vi "Set_Horizontal_ROI.vi"(8 "error in (no error)":errorcluster, 10 "input cluster":T1={"Mode"=enum."ROI", "Manual LUT"={"Minimum"=0.0, "Maximum"=0.0}, "ImageProcessed"=refnum, "Image "=refnum, "Log?"=FALSE, "Auto?"=FALSE, "ROI"={"Global Rectangle"=[], "Contours"=[]}, "ROI Parameters"={"Count"=0.0, "Size(um)"=0.0}, "Image X"=0, "Image Y"=0, "Horizontal ROI"={"Global Rectangle"=[], "Contours"=[]}, "HROI Pos"=0, "Custom ROI"={"Global Rectangle"=[], "Contours"=[]}, "Intensity Graph"=[], "Image Type"=7} {"Image Type" items=["Grayscale (U8)", "Grayscale (U16)"]; "ROI Parameters"."Size(um)" min=0 max=255 step=0.1 format="%.2f"; "ROI Parameters"."Count" min=0 max=255 step=0.1 format="%.2f"}) -> (0 "error out":errorcluster, 2 "output cluster":T1={"Mode"=enum."ROI", "Manual LUT"={"Minimum"=0.0, "Maximum"=0.0}, "ImageProcessed"=refnum, "Image "=refnum, "Log?"=FALSE, "Auto?"=FALSE, "ROI"={"Global Rectangle"=[], "Contours"=[]}, "ROI Parameters"={"Count"=0.0, "Size(um)"=0.0}, "Image X"=0, "Image Y"=0, "Horizontal ROI"={"Global Rectangle"=[], "Contours"=[]}, "HROI Pos"=0, "Custom ROI"={"Global Rectangle"=[], "Contours"=[]}, "Intensity Graph"=[], "Image Type"=7} {"Image Type" items=["Grayscale (U8)", "Grayscale (U16)"]; "ROI Parameters"."Size(um)" min=0 max=255 step=0.1 format="%.2f"; "ROI Parameters"."Count" min=0 max=255 step=0.1 format="%.2f"})   [LabVIEW 2023, in "Camera_Controller.lvlib"]
uses:
  Camera_Controller.lvlib
  typedefs/ImageProcessingParameters.ctl
  <vilib>/vision/Image Controls.llb/IMAQ Image.ctl
  typedefs/Image Type.ctl
  <vilib>/vision/NI_Vision_Development_Module.lvlib
  typedefs/typedefs.lvlib
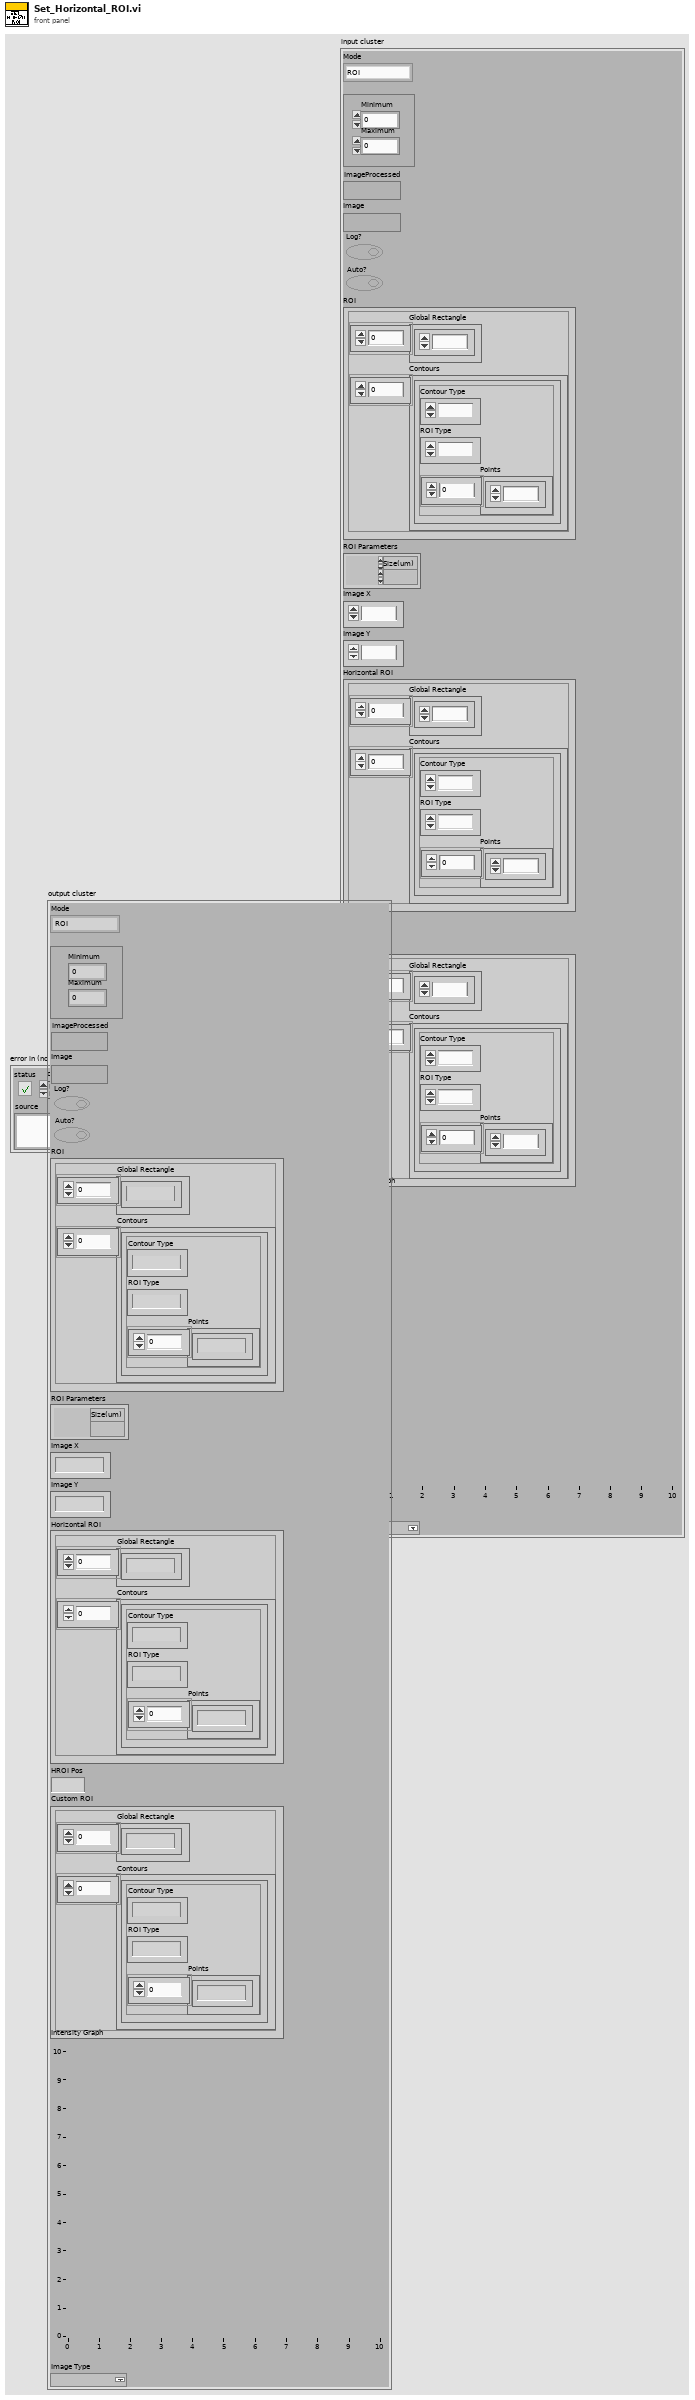
[diagram p1: front panel]
types:
  T1 = typedef "typedefs.lvlib/ImageProcessingParameters.ctl" = cluster{"Mode":enum16{"ROI", "Image"}, "Manual LUT":cluster{"Minimum":dbl, "Maximum":dbl}, "ImageProcessed":T2, "Image ":T2, "Log?":bool, "Auto?":bool, "ROI":cluster{"Global Rectangle":i32[], "Contours":cluster{"Contour Type":u32, "ROI Type":u32, "Points":i32[]}[]}, "ROI Parameters":cluster{"Count":sgl, "Size(um)":sgl}, "Image X":i32, "Image Y":i32, "Horizontal ROI":cluster{"Global Rectangle":i32[], "Contours":cluster{"Contour Type":u32, "ROI Type":u32, "Points":i32[]}[]}, "HROI Pos":u16, "Custom ROI":cluster{"Global Rectangle":i32[], "Contours":cluster{"Contour Type":u32, "ROI Type":u32, "Points":i32[]}[]}, "Intensity Graph":u8[][], "Image Type":T3}
  T2 = typedef "IMAQ Image.ctl" = refnum<image>
  T3 = typedef "typedefs.lvlib/Image Type.ctl" = u32
  T4 = cluster{"x1Left":i32, "y1Top":i32, "x2Right":i32, "y2Bottom":i32}
  T5 = typedef "ROI Descriptor" = cluster{"Global Rectangle":i32[], "Contours":cluster{"ID":enum32{"External", "Internal"}, "Type":u32, "Coordinates":i32[]}[]}
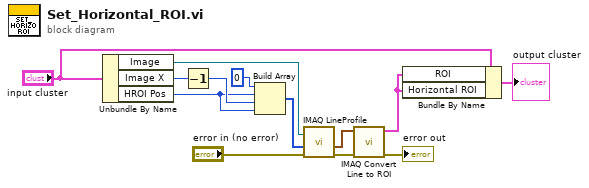
[diagram p0: block diagram]
diagram:
  n1 = Unbundle By Name("input cluster") -> ("Image"=w9:T2, "Image X"=w5:i32, "HROI Pos"=w2:u16)
  n2 = Decrement(x=w5) -> (x-1=w4:i32)
  n3 = Build Array(u16 0 ("element"), w2, w4, w2) -> (w6:i32[])
  n4 = call "IMAQ LineProfile"("error in (no error)"="error in (no error)", "Line Coordinates"=w6, "Image"=w9) -> ("Global Rectangle"=w1:T4, "error out"=w13:errorcluster)  [unwired: 2 in, 2 out]
  n5 = call "IMAQ Convert Line to ROI"("error in (no error)"=w13, "Line"=w1) -> ("error out"=→"error out":errorcluster, "ROI Descriptor"=w3:T5)  [unwired: 7 in]
  n6 = Bundle By Name(cluster="input cluster", "ROI"=w3, "Horizontal ROI"=w3) -> (→"output cluster":T1)
